vi "MeasAction.vi"(8 "error in (no error)":errorcluster caption="entrée d'erreur (pas d'erreur)", 9 "CurvePointIndex":i32, 10 "AllPointIndex":i32, 11 "InstrClassIn":refnum<class "KlingerMotor.lvclass"> caption="DNL_LabVIEW Object in") -> (0 "error out":errorcluster caption="sortie d'erreur", 2 "MeasDatOut":dbl[](array[numeric]), 3 "InstrClassOut":refnum<class "KlingerMotor.lvclass"> caption="DNL_LabVIEW Object out")   [LabVIEW 2019, in "KlingerMotor.lvclass"]
uses:
  KlingerMotor.lvclass
  C:/Programmes Labview/LabScanV1A/DevicesClass/BaseDevice/BaseDevice.lvclass
  KlingerMotor.lvclass/KlingerMotor.ctl
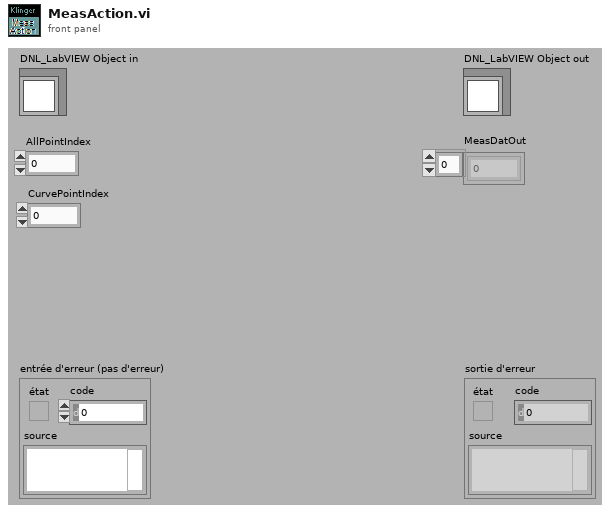
[diagram p1: front panel]
types:
  T1 = typedef "KlingerMotor.lvclass/KlingerMotor_Func.ctl" = enum16{"Positions (mm)", "Position (ps)", "ReadWPos (ps)", "ReadWPos (mm)", "ReadZPos (ps)", "ReadZPos (mm)"}
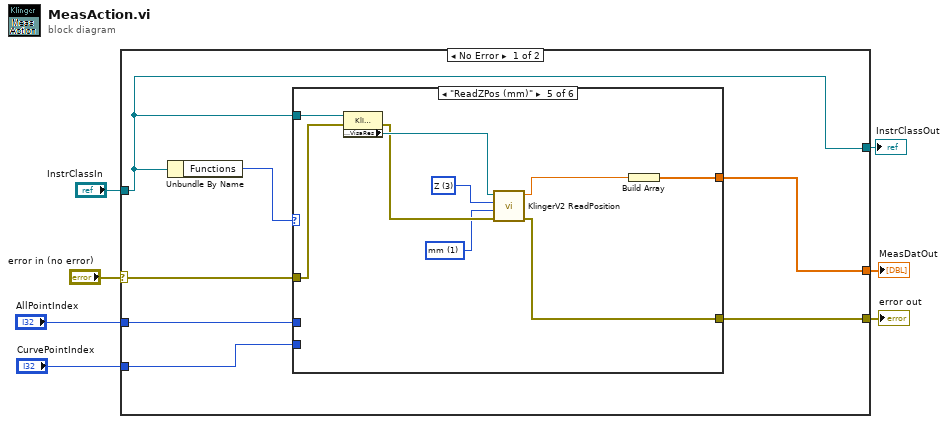
[diagram p0: block diagram]
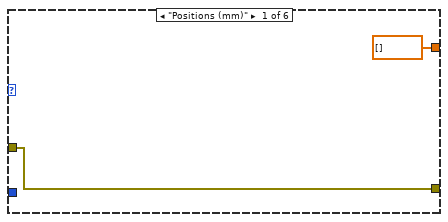
[diagram p2: hidden frame]
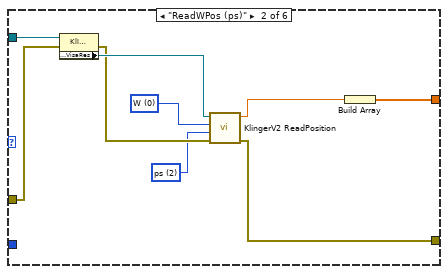
[diagram p3: hidden frame]
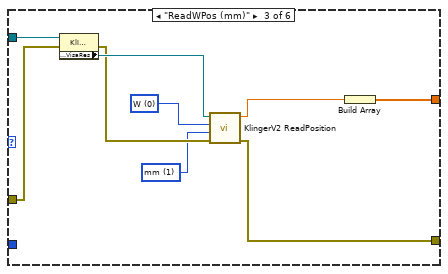
[diagram p4: hidden frame]
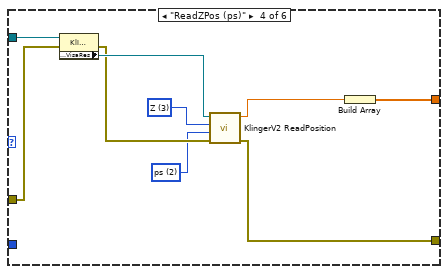
[diagram p5: hidden frame]
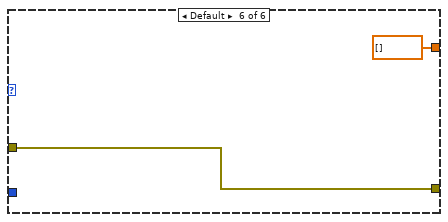
[diagram p6: hidden frame]
diagram:
  n1 = case shown="No Error" "error in (no error)" {
    selector: "error in (no error)" -> [w10 w55]
    tunnel: "InstrClassIn" -> [w8 w56]
    tunnel: [w8 w56] -> w5
    tunnel: "AllPointIndex" -> [w14 _]
    tunnel: [w13 w55] -> w3
    tunnel: [w12 _] -> w2
    tunnel: "CurvePointIndex" -> [w9 _]
    frame No Error {
      n2 = Unbundle By Name(w8) -> ("Functions"=w11:T1)
      n3 = case shown="\"ReadZPos (mm)\"" w11 {
        tunnel: w14 -> [_ _ _ _ _ _]
        tunnel: [w16 w18 w27 w36 w45 w53] -> w13
        tunnel: [dbl[] [] ("Outputs") w19 w28 w37 w46 dbl[] [] ("Outputs")] -> w12
        tunnel: w10 -> [w16 w23 w32 w41 w50 w53]
        tunnel: w9 -> [_ _ _ _ _ _]
        tunnel: w8 -> [_ w25 w34 w43 w52 _]
        frame "Positions (mm)" {
        }
        frame "ReadWPos (ps)" {
          w17 = u8 0 items=["W", "X", "Y", "Z"] ("Axe")
          w21 = u8 2 items=["Pas", "mm", "ps", "Degré (°)"] ("UnitDem")
          n4 = property class="KlingerMotor.lvclass"(reference=w25, error in=w23) -> (error out=w22:errorcluster, "Accessor:VisaRes"=w24:refnum<visa-resource-name>)  [unwired: 1 out]
          n5 = call <userlib>:"KlingerV2 ReadPosition.vi"("error in"=w22, "UnitDem"=w21, "Axe"=w17, "VISA Rsrc"=w24) -> ("error out"=w18:errorcluster, "Position"=w20:dbl)  [unwired: 1 in, 5 out]
          n6 = Build Array(w20) -> (w19:dbl[])
        }
        frame "ReadWPos (mm)" {
          w26 = u8 0 items=["W", "X", "Y", "Z"] ("Axe")
          w30 = u8 1 items=["Pas", "mm", "ps", "Degré (°)"] ("UnitDem")
          n7 = property class="KlingerMotor.lvclass"(reference=w34, error in=w32) -> (error out=w31:errorcluster, "Accessor:VisaRes"=w33:refnum<visa-resource-name>)  [unwired: 1 out]
          n8 = call <userlib>:"KlingerV2 ReadPosition.vi"("error in"=w31, "UnitDem"=w30, "Axe"=w26, "VISA Rsrc"=w33) -> ("error out"=w27:errorcluster, "Position"=w29:dbl)  [unwired: 1 in, 5 out]
          n9 = Build Array(w29) -> (w28:dbl[])
        }
        frame "ReadZPos (ps)" {
          w35 = u8 3 items=["W", "X", "Y", "Z"] ("Axe")
          w39 = u8 2 items=["Pas", "mm", "ps", "Degré (°)"] ("UnitDem")
          n10 = property class="KlingerMotor.lvclass"(reference=w43, error in=w41) -> (error out=w40:errorcluster, "Accessor:VisaRes"=w42:refnum<visa-resource-name>)  [unwired: 1 out]
          n11 = call <userlib>:"KlingerV2 ReadPosition.vi"("error in"=w40, "UnitDem"=w39, "Axe"=w35, "VISA Rsrc"=w42) -> ("error out"=w36:errorcluster, "Position"=w38:dbl)  [unwired: 1 in, 5 out]
          n12 = Build Array(w38) -> (w37:dbl[])
        }
        frame "ReadZPos (mm)" {
          w44 = u8 3 items=["W", "X", "Y", "Z"] ("Axe")
          w48 = u8 1 items=["Pas", "mm", "ps", "Degré (°)"] ("UnitDem")
          n13 = property class="KlingerMotor.lvclass"(reference=w52, error in=w50) -> (error out=w49:errorcluster, "Accessor:VisaRes"=w51:refnum<visa-resource-name>)  [unwired: 1 out]
          n14 = call <userlib>:"KlingerV2 ReadPosition.vi"("error in"=w49, "UnitDem"=w48, "Axe"=w44, "VISA Rsrc"=w51) -> ("error out"=w45:errorcluster, "Position"=w47:dbl)  [unwired: 1 in, 5 out]
          n15 = Build Array(w47) -> (w46:dbl[])
        }
        frame Default {
        }
      }
    }
    frame Error {
    }
  }
  "error out" <- w3
  "InstrClassOut" <- w5
  "MeasDatOut" <- w2
